vi "Read Parent.vi"(8 "Error In":errorcluster, 11 "Abstract In":refnum<class "Abstract.lvclass">) -> (0 "Error Out":errorcluster, 2 "Parent":refnum<class "Abstract.lvclass">, 3 "Abstract Out":refnum<class "Abstract.lvclass">)   [LabVIEW 2018, in "Toolkit.lvlib" / "Nodes.lvlib" / "Abstract.lvclass"]
uses:
  Abstract.lvclass
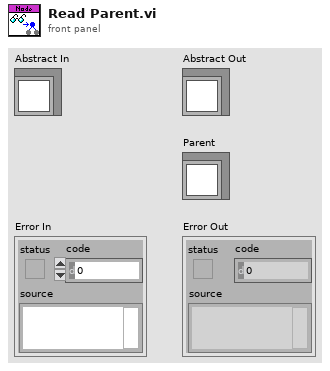
[diagram p1: front panel]
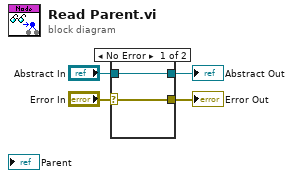
[diagram p0: block diagram]
diagram:
  n1 = case shown="No Error" "Error In" {
    selector: "Error In" -> [w5 w8]
    tunnel: [w5 w8] -> w3
    tunnel: [w6 w7] -> w1
    tunnel: "Abstract In" -> [w6 w7]
    frame No Error {
    }
    frame Error {
    }
  }
  "Error Out" <- w3
  "Abstract Out" <- w1
